vi "Monitor HW.vi"(8 "error in (no error)":errorcluster, 9 "Stage Data Class":refnum<data-value>, 10 "Y-Axis":refnum<class "iMotion Controller.lvclass">, 11 "X Axis":refnum<class "iMotion Controller.lvclass">) -> ()   [LabVIEW 2022 SP3, in "XY Stage Process.lvlib" / "XY Stage Process.lvclass"]
uses:
  XY Stage Process.lvclass
  XY Stage Process.lvclass/XY Stage Process.ctl
  XY Stage Data Class/XY Stage Data Class.lvclass
  Axis Objects/iMotion Controller/iMotion Controller.lvclass
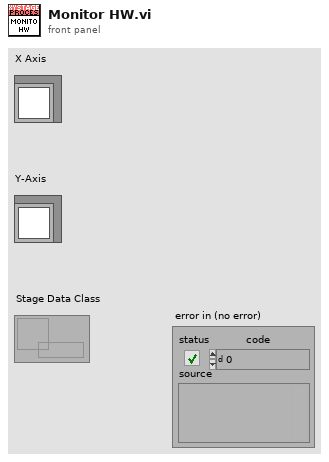
[diagram p1: front panel]
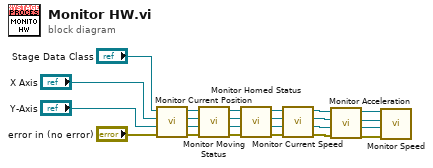
[diagram p0: block diagram]
diagram:
  n1 = call "Monitor Current Position.vi"("error in (no error)"="error in (no error)", "Y-Axis In"="Y-Axis", "X-Axis In"="X Axis", "Stage Data Class"="Stage Data Class") -> ("error out"=w13:errorcluster, "Y-Axis Out"=w16:refnum<class "iMotion Controller.lvclass">, "X-Axis Out"=w17:refnum<class "iMotion Controller.lvclass">, "Stage Data Class"=w19:refnum<data-value>)  [unwired: 4 in]
  n2 = call "Monitor Moving Status.vi"("error in (no error)"=w13, "YAxis In"=w16, "X-Axis In"=w17, "Stage Data Class in"=w19) -> ("error out"=w24:errorcluster, "Y-Axis Out"=w21:refnum<class "iMotion Controller.lvclass">, "X-Axis Out"=w22:refnum<class "iMotion Controller.lvclass">, "Stage Data Class out"=w23:refnum<data-value>)  [unwired: 4 in]
  n3 = call "Monitor Homed Status.vi"("error in (no error)"=w24, "Y-Axis In"=w21, "X-Axis In"=w22, "Stage Data Class"=w23) -> ("error out"=w9:errorcluster, "Y-Axis Out"=w10:refnum<class "iMotion Controller.lvclass">, "X-Axis Out"=w11:refnum<class "iMotion Controller.lvclass">, "Stage Data Class"=w12:refnum<data-value>)  [unwired: 4 in]
  n4 = call "Monitor Current Speed.vi"("error in (no error)"=w9, "Y-Axis In"=w10, "X-Axis In"=w11, "Stage Data Class"=w12) -> ("error out"=w5:errorcluster, "Y-Axis Out"=w6:refnum<class "iMotion Controller.lvclass">, "X-Axis Out"=w7:refnum<class "iMotion Controller.lvclass">, "Stage Data Class"=w8:refnum<data-value>)  [unwired: 4 in]
  n5 = call "Monitor Acceleration.vi"("error in (no error)"=w5, "Y-Axis In"=w6, "X-Axis In"=w7, "Stage Data Class"=w8) -> ("error out"=w1:errorcluster, "Y-Axis Out"=w2:refnum<class "iMotion Controller.lvclass">, "X-Axis Out"=w3:refnum<class "iMotion Controller.lvclass">, "Stage Data Class"=w4:refnum<data-value>)  [unwired: 4 in]
  n6 = call "Monitor Speed.vi"("error in (no error)"=w1, "Y-Axis In"=w2, "X-Axis In"=w3, "Stage Data Class"=w4) -> ()  [unwired: 4 in, 4 out]
